vi "PlotRxPower.vi"(1 "SHOW PLOT(T)":bool, 11 "error in (no error)":errorcluster, 12 "GET FROM FILE(T)":bool, 13 "CF(MHZ)":dbl=10.0 min=0.0 max=150.0 format="%#_13g", 14 "BW(MHZ)":dbl=10.0 format="%#_13g") -> (2 "band (dbfs/mhz)":dbl[](array[numeric]), 3 "peak (dbfs/mhz)":dbl[](array[numeric]), 15 "error out":errorcluster)   [LabVIEW 2018]
panel:
  out "time(s)":dbl
  out "start(s)":dbl format="%_19f"
  in  "selected path":path
  in  "Use Static File Path":bool
  in  "GET FILE PATH":path=path "C:/Users/ThomasWattson/TomWOneDrive/OneDrive - Rage Systems/Documents - Tetra/Test Docs/Test Results/WAM/Prototype SN20-29/7-7-21"
  out "command":string
  out "console  output":string
  # "Input Dialog. Check \"Show Plot\" if desired"
  # "File Path Dialog. Check if file save desired"
  # "Band  & Peak Power Outputs"
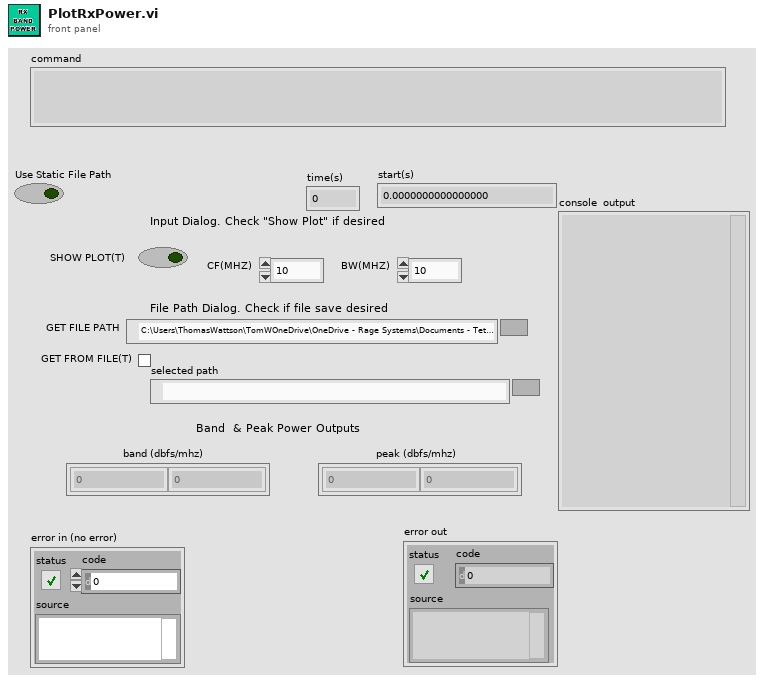
[diagram p1: front panel]
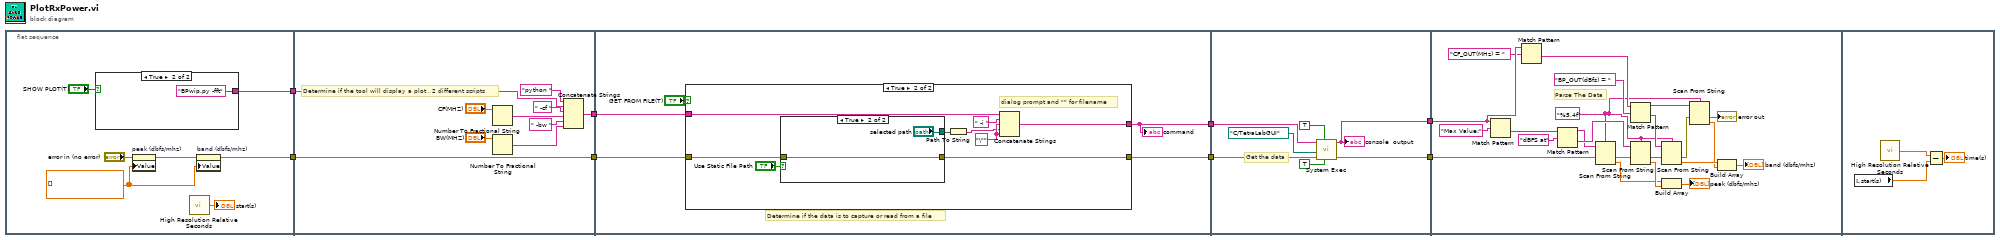
[diagram p0: block diagram]
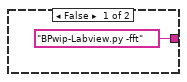
[diagram p2: hidden frame]
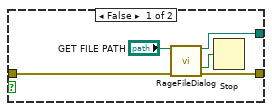
[diagram p4: hidden frame]
diagram:
  n1 = flat-sequence {
    tunnel: [w14] -> w5
    tunnel: [w10] -> w4
    tunnel: [w21] -> w7
    tunnel: w5 -> [w19]
    tunnel: w4 -> [w18]
    tunnel: [w18] -> w3
    tunnel: w7 -> [w31]
    tunnel: [w30] -> w6
    tunnel: w3 -> [w29]
    tunnel: [w28] -> w2
    tunnel: [w57] -> w8
    tunnel: w6 -> [w56]
    tunnel: w2 -> [w55]
    tunnel: [w51] -> w1
    tunnel: w8 -> [w80]
    tunnel: w1 -> [w62]
    frame #0 {
      w11 = dbl[] [] ("peak (dbfs/mhz)")
      n2 = case shown="True" "SHOW PLOT(T)" {
        tunnel: ["BPwip-Labview.py -fft" ("command line") "BPwip.py -fft" ("command line")] -> w14
        frame False {
        }
        frame True {
        }
      }
      n3 = property on="peak (dbfs/mhz)" class="Arr (strict)"(error in="error in (no error)", "Value"=w11) -> (error out=w13:errorcluster)  [unwired: 1 in, 1 out]
      n4 = call <vilib>:"High Resolution Relative Seconds.vi"() -> ("relative seconds"=→"start(s)":dbl)
      n5 = property on="band (dbfs/mhz)" class="Arr (strict)"(error in=w13, "Value"=w11) -> (error out=w10:errorcluster)  [unwired: 1 in, 1 out]
    }
    frame #1 {
      # "Determine if the tool will display a plot . 2 different scripts"
      n6 = Number To Fractional String(number="CF(MHZ)") -> (F-format string=w27:string)  [unwired: 3 in]
      n7 = Number To Fractional String(number="BW(MHZ)") -> (F-format string=w20:string)  [unwired: 3 in]
      n8 = Concatenate Strings("python " ("string"), w19, " -cf " ("string"), w27, " -bw " ("string"), w20) -> (w21:string)
    }
    frame #2 {
      # "Determine if the data is to capture or read from a file"
      n9 = case shown="True" "GET FROM FILE(T)" {
        tunnel: [w34 w41] -> w30
        tunnel: w31 -> [w34 w38]
        tunnel: w29 -> [w33 w37]
        tunnel: [w33 w36] -> w28
        frame False {
          # "dialog prompt and \"\" for filename"
        }
        frame True {
          w42 = "\"" ("string")
          # "dialog prompt and \"\" for filename"
          n10 = case shown="True" "Use Static File Path" {
            tunnel: [w47 "selected path"] -> w40
            tunnel: w37 -> [w45 w49]
            tunnel: [w44 w49] -> w36
            frame False {
              n11 = call "RageFileDialog.vi"("start path"="GET FILE PATH", "error in"=w45) -> ("selected path"=w47:path, "cancelled"=w48:bool, "error out"=w44:errorcluster)  [unwired: 10 in, 1 out]
              n12 = Stop(stop? (T)=w48) -> ()
            }
            frame True {
            }
          }
          n13 = Path To String(path=w40) -> (string=w39:string)
          n14 = Concatenate Strings(w38, " -i " ("string"), w42, w39, w42) -> (w41:string)
        }
      }
      "command" <- w30
    }
    frame #3 {
      # "Get the data"
      n15 = call <vilib>:"System Exec.vi"("run minimized? (F)"=TRUE, "wait until completion? (T)"=TRUE, "error in (no error)"=w55, "working directory"=path "C:/TetraLabGUI", "command line"=w56) -> ("error out"=w51:errorcluster, "standard output"=w57:string)  [unwired: 3 in, 2 out]
      "console  output" <- w57
    }
    frame #4 {
      w67 = "%5.4f" ("format string")
      # "Parse The Data"
      n16 = Match Pattern(string=w80, regular expression="Max Value:") -> (after substring=w73:string)  [unwired: 1 in, 3 out]
      n17 = Match Pattern(string=w80, regular expression="CF_OUT(MHz) = ") -> (after substring=w70:string)  [unwired: 1 in, 3 out]
      n18 = Match Pattern(string=w73, regular expression="dBFS at") -> (before substring=w74:string, after substring=w75:string)  [unwired: 1 in, 2 out]
      n19 = Scan From String(format string=w67, input string=w74, error in=w62) -> (error out=w61:errorcluster, output 1=w77:dbl)  [unwired: 2 in, 2 out]
      n20 = Match Pattern(string=w70, regular expression="BP_OUT(dBfs) = ") -> (before substring=w69:string, after substring=w68:string)  [unwired: 1 in, 2 out]
      n21 = Scan From String(format string=w67, input string=w75, error in=w61) -> (error out=w60:errorcluster, output 1=w78:dbl)  [unwired: 2 in, 2 out]
      n22 = Scan From String(format string=w67, input string=w68, error in=w60) -> (error out=w59:errorcluster, output 1=w65:dbl)  [unwired: 2 in, 2 out]
      n23 = Build Array(w77, w78) -> (→"peak (dbfs/mhz)":dbl[])
      n24 = Scan From String(format string=w67, input string=w69, error in=w59) -> (error out=→"error out":errorcluster, output 1=w64:dbl)  [unwired: 2 in, 2 out]
      n25 = Build Array(w65, w64) -> (→"band (dbfs/mhz)":dbl[])
    }
    frame #5 {
      n26 = local read "start(s)"() -> (w82:dbl)
      n27 = call <vilib>:"High Resolution Relative Seconds.vi"() -> ("relative seconds"=w83:dbl)
      n28 = Subtract(x=w83, y=w82) -> (x-y=→"time(s)":dbl)
    }
  }
